vi "LoadUnflattenClassData.vi"(8 "error in":errorcluster, 10 "Class Data File Path":path, 11 "TestCase in":refnum<class "TestCase.lvclass">) -> (0 "error out":errorcluster, 3 "TestCase out":refnum<class "TestCase.lvclass">)   [LabVIEW 2027, in "VeriStandTestUtilities.lvlib"]
uses:
  VeriStandTestUtilities.lvlib
  <vilib>/addons/_JKI Toolkits/VI Tester/TestCase.llb/TestCase.lvclass
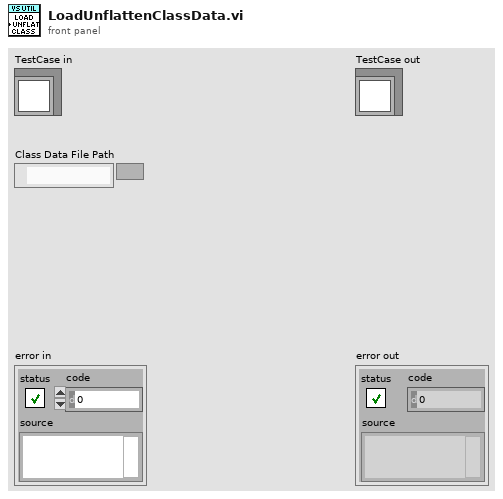
[diagram p1: front panel]
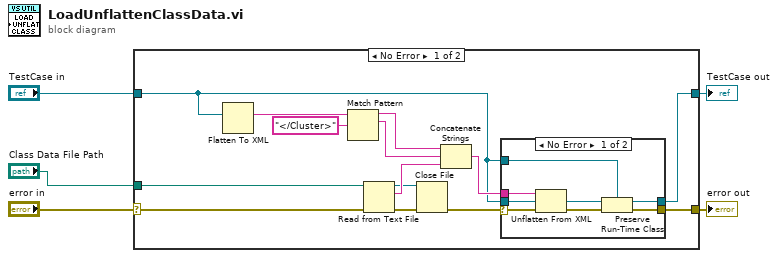
[diagram p0: block diagram]
diagram:
  n1 = case shown="No Error" "error in" {
    selector: "error in" -> [w15 w30]
    tunnel: [w9 w31] -> w2
    tunnel: "TestCase in" -> [w7 w31]
    tunnel: [w10 w30] -> w4
    tunnel: "Class Data File Path" -> [w6 _]
    frame No Error {
      n2 = Flatten To XML(6:w7) -> (2:w19:string)
      n3 = Match Pattern(string=w19, regular expression="</Cluster>") -> (before substring=w17:string, match substring=w16:string)  [unwired: 1 in, 2 out]
      n4 = Read from Text File(file (use dialog)=w6, error in=w15) -> (refnum out=w12:refnum<file>, text=w14:string, error out=w13:errorcluster)  [unwired: 2 in, 1 out]
      n5 = Close File(refnum=w12, error in=w13) -> (error out=w11:errorcluster)  [unwired: 1 out]
      n6 = Concatenate Strings(w17, w16, w14) -> (w8:string)
      n7 = case shown="No Error" w11 {
        selector: w11 -> [w27 w29]
        tunnel: [w20 w29] -> w10
        tunnel: w7 -> [w26 w28]
        tunnel: [w22 w28] -> w9
        tunnel: w8 -> [w25 _]
        tunnel: w7 -> [w24 _]
        frame No Error {
          n8 = Unflatten From XML(xml string=w25, type=w26, error in (no error)=w27) -> (value=w23:refnum<class "TestCase.lvclass">, error out=w21:errorcluster)
          n9 = Preserve Run-Time Class(object in=w23, error in=w21, 2:w24) -> (object out=w22:refnum<class "TestCase.lvclass">, error out=w20:errorcluster)
        }
        frame Error {
        }
      }
    }
    frame Error {
    }
  }
  "error out" <- w4
  "TestCase out" <- w2
